vi "AuMT8852B Tester Page Scan Repetition Mode.vi"(5 "Mode (R1)":u16(ring) items=["R0", "R1", "R2"], 7 "Set/Get (Set)":enum16{"Set", "Get"}(ring), 8 "error in (no error)":errorcluster, 11 "VISA session":refnum<visa-resource-name>) -> (0 "error out":errorcluster, 2 "error code":i32, 3 "VISA session out":refnum<visa-resource-name>, 4 "Mode out":u16(ring) items=["R0", "R1", "R2"])   [LabVIEW 2017]
doc: "Anritsu MT8852B Bluetooth Tester\n\nControls the EUT page scan repetition mode.\n\nINPUTS\nSet/Get - whether the value is being sent to or retrieved from the instrument.\nMode - sets the mode to be used by the tester.\n\nOUTPUTS\nMode out - the mode currently in use by the tester."
uses:
  <instrlib>/aumt8852B/General/Utilities/MT8850 Attribute ID.ctl
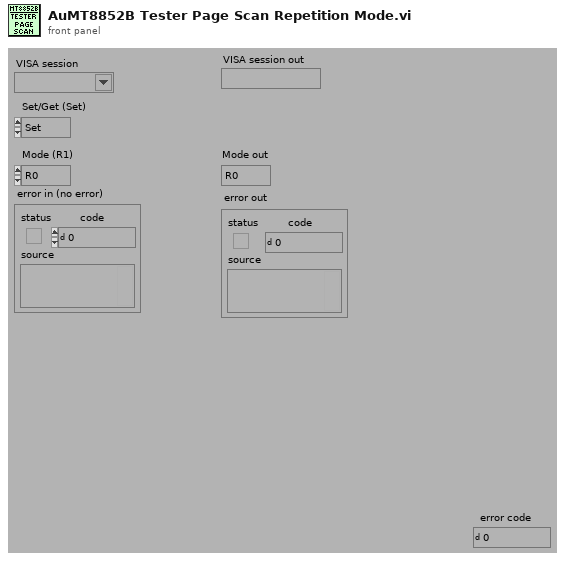
[diagram p1: front panel]
types:
  T1 = typedef "MT8850 Attribute ID.ctl" = enum16{"Operation mode", "Selected script", "EUT address source", "EUT Address", "EUT HCI RS232 Baud Rate", "Tester GPIB Address", "Tester RS232 Baud Rate", "Tester Bluetooth Address", "Tester Contrast", "Tester Key Click On", "Tester Modulation Index", "Tester Poll-Null Mode", "Tester Power Range", "Tester RS232 Mode", "Beep on Illegal Entry", "Display User Text", "User Text", "Calibration TX Modulation DAC", "Calibration RX Channel", "Calibration TX Channel", "Calibration TX Power", "Calibration Use TX Table", "Inquiry Request User-friendly Name", "Inquiry Number of Responses", "Inquiry Timeout", "Script Frequency Display", "Script Loop Count", "Script Loop Continuously", "Script Loop Stop on Fail", "Link timeout", "Page timeout", "Filter bandwidth", "SCO air code", "SCO bit position", "SCO input code", "SCO input data", "SCO input sample size", "SCO loopback mode", "SCO packet type", "SCO tone generator", "Tester page scan repetition mode", "Tester follow test mode", "Tester authentication state", "Tester authentication pin code", "Tester authentication pin length"}
  T2 = typedef "Attribute Status.ctl" = enum16{"No I/O needed", "I/O needed"}
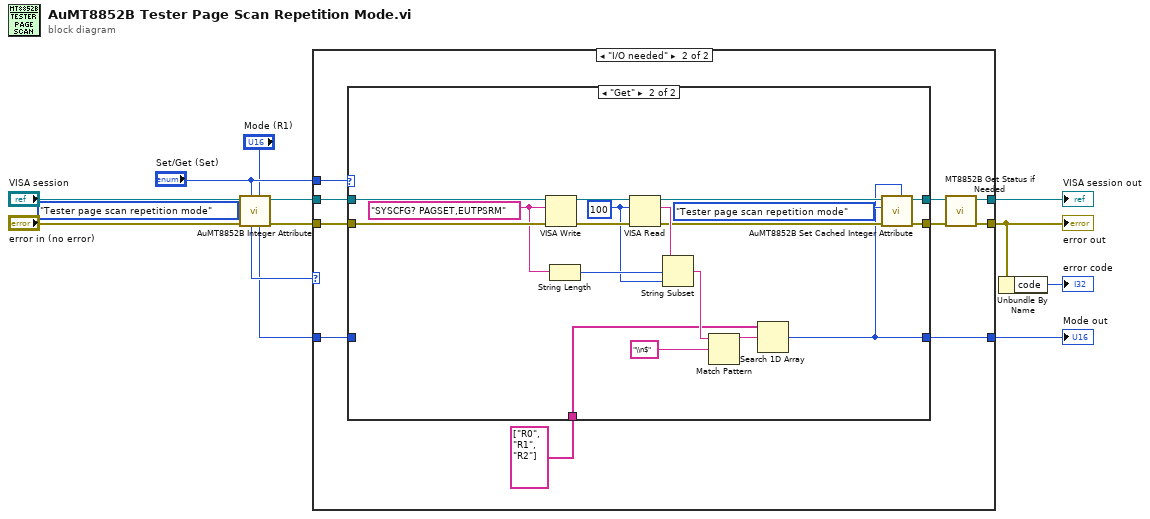
[diagram p0: block diagram]
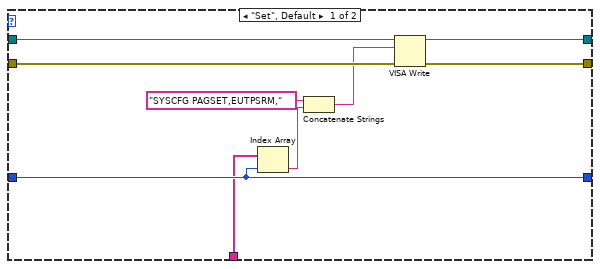
[diagram p3: hidden frame]
diagram:
  n1 = call <instrlib>:"AuMT8852B Integer Attribute.vi"("Value (0)"="Mode (R1)", "Set/Get (Set)"="Set/Get (Set)", "error in (no error)"="error in (no error)", "Attribute ID"=MT8850_Attribute_ID."Tester page scan repetition mode", "VISA session"="VISA session") -> ("error out"=w9:errorcluster, "VISA session out"=w8:refnum<visa-resource-name>, "Value out"=w3:i32, "Status"=w6:T2)  [unwired: 3 in]
  n2 = case shown="\"I/O needed\"" w6 {
    tunnel: w8 -> [w16 w25]
    tunnel: [w16 w23] -> w13
    tunnel: w9 -> [w15 w24]
    tunnel: [w15 w22] -> w2
    tunnel: "Set/Get (Set)" -> [_ w26]
    tunnel: w3 -> [w14 w19]
    tunnel: [w14 w18] -> w12
    frame "No I/O needed" {
    }
    frame "I/O needed" {
      n3 = case shown="\"Get\"" w26 {
        tunnel: w25 -> [w33 w53]
        tunnel: w24 -> [w32 w51]
        tunnel: [w35 w40] -> w21
        tunnel: [w34 w41] -> w20
        tunnel: w19 -> [w28 _]
        tunnel: [w28 w36] -> w18
        tunnel: string[] ["R0", "R1", "R2"] -> [w27 w43]
        frame "Set", Default {
          n4 = Index Array(array=w27, index=w28) -> (element=w29:string)
          n5 = Concatenate Strings("SYSCFG PAGSET,EUTPSRM," ("string"), w29) -> (w31:string)
          n6 = VISA Write(VISA resource name=w33, write buffer=w31, error in (no error)=w32) -> (VISA resource name out=w35:refnum<visa-resource-name>, error out=w34:errorcluster)  [unwired: 1 out]
        }
        frame "Get" {
          w47 = u32 100 ("byte count (0)")
          w49 = "SYSCFG? PAGSET,EUTPSRM" ("write buffer (\"\")")
          n7 = VISA Write(VISA resource name=w53, write buffer=w49, error in (no error)=w51) -> (VISA resource name out=w52:refnum<visa-resource-name>, error out=w50:errorcluster)  [unwired: 1 out]
          n8 = String Length(string=w49) -> (length=w48:i32)
          n9 = VISA Read(VISA resource name=w52, byte count=w47, error in (no error)=w50) -> (VISA resource name out=w38:refnum<visa-resource-name>, read buffer=w46:string, error out=w39:errorcluster)  [unwired: 1 out]
          n10 = String Subset(string=w46, offset (0)=w48, length (rest)=w47) -> (substring=w45:string)
          n11 = Match Pattern(string=w45, regular expression="\\n$") -> (before substring=w44:string)  [unwired: 1 in, 3 out]
          n12 = Search 1D Array(1D array=w43, element=w44) -> (index of element=w36:i32)  [unwired: 1 in]
          n13 = call <instrlib>:"AuMT8852B Set Cached Integer Attribute.vi"("Value (0)"=w36, "error in (no error)"=w39, "Attribute ID"=MT8850_Attribute_ID."Tester page scan repetition mode", "VISA session"=w38) -> ("error out"=w41:errorcluster, "VISA session out"=w40:refnum<visa-resource-name>)  [unwired: 6 in]
        }
      }
      n14 = call <instrlib>:"MT8852B Get Status if Needed.vi"("error in (no error)"=w20, "VISA session"=w21) -> ("error out"=w22:errorcluster, "VISA session out"=w23:refnum<visa-resource-name>)  [unwired: 8 in]
    }
  }
  "error out" <- w2
  "VISA session out" <- w13
  "Mode out" <- w12
  n15 = Unbundle By Name(w2) -> ("code"=→"error code":i32)
